vi "Main.vi"   [LabVIEW 2020]
uses:
  PreStep/PreStep.lvclass
  C:/Users/SAS/Desktop/Decorator/Base Decorator/Base Decorator.lvclass
  C:/Users/SAS/Desktop/Decorator/Testable/Testable.lvclass
  Another Concrete Step/Another Concrete Step.lvclass
  PostStep/PostStep.lvclass
  Concrete Test step/Concrete Test Step.lvclass
  LogDB/LogDB.lvclass
  LogFile/LogFile.lvclass
  Base Decorator/Base Decorator.lvclass
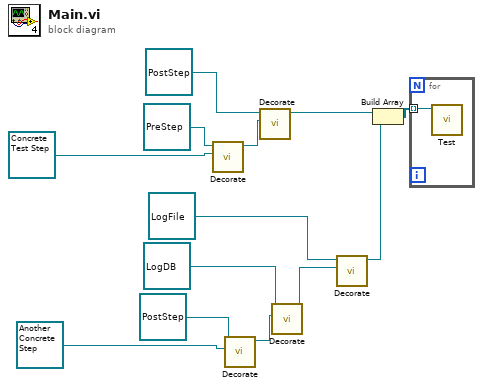
[diagram p0: block diagram]
diagram:
  n1 = call "Decorate.vi"("To be decorated"=refnum<class "Concrete Test Step.lvclass"> refnum ("Concrete Test Step.lvclass"), "Base Decorator in"=refnum<class "PreStep.lvclass"> refnum ("PreStep.lvclass")) -> ("Base Decorator out"=w10:refnum<class "PreStep.lvclass">)  [unwired: 8 in, 1 out]
  n2 = call "Decorate.vi"("To be decorated"=refnum<class "Another Concrete Step.lvclass"> refnum ("Another Concrete Step.lvclass"), "Base Decorator in"=refnum<class "PostStep.lvclass"> refnum ("PostStep.lvclass")) -> ("Base Decorator out"=w8:refnum<class "PostStep.lvclass">)  [unwired: 8 in, 1 out]
  n3 = call "Decorate.vi"("To be decorated"=w10, "Base Decorator in"=refnum<class "PostStep.lvclass"> refnum ("PostStep.lvclass")) -> ("Base Decorator out"=w9:refnum<class "PostStep.lvclass">)  [unwired: 8 in, 1 out]
  n4 = call "Decorate.vi"("To be decorated"=w8, "Base Decorator in"=refnum<class "LogDB.lvclass"> refnum ("LogDB.lvclass")) -> ("Base Decorator out"=w1:refnum<class "LogDB.lvclass">)  [unwired: 8 in, 1 out]
  n5 = call "Decorate.vi"("To be decorated"=w1, "Base Decorator in"=refnum<class "LogFile.lvclass"> refnum ("LogFile.lvclass")) -> ("Base Decorator out"=w3:refnum<class "LogFile.lvclass">)  [unwired: 8 in, 1 out]
  n6 = Build Array(w9, w3) -> (w13:refnum<class "Base Decorator.lvclass">[])
  n7 = for {
    tunnel: w13 -> [w14] mode=indexing
    n8 = call-dynamic "Test.vi"("Base Decorator in"=w14) -> ()  [unwired: 8 in, 3 out]
  }
